vi "centerFilter.vi"(0 "Image In":T2, 1 "Color Mode (Color Threshold 1)":u16(ring) items=["RGB", "HSL", "HSV", "HSI"], 2 "Red or Hue Range (Color Threshold 1)":cluster{"Lower value":i32, "Upper value":i32}={"Lower value"=0, "Upper value"=12}, 3 "Green or Sat Range (Color Threshold 1)":cluster{"Lower value":i32, "Upper value":i32}={"Lower value"=24, "Upper value"=255}, 5 "Blue\nBlue or Sat Range (Color Threshold 1)":cluster{"Lower value":i32, "Upper value":i32}={"Lower value"=24, "Upper value"=255}, 7 "error in":errorcluster) -> (20 "Image Out":T2, 21 "Centroid (Centroid 1)":cluster{"X Centroid":sgl, "Y Centroid":sgl} {"Y Centroid" format="%.2f"; "X Centroid" format="%.2f"}, 22 "Calibrated Centroid (Centroid 1)":cluster{"X Centroid":sgl, "Y Centroid":sgl} {"Y Centroid" format="%.2f"; "X Centroid" format="%.2f"}, 23 "Particle Reports (Pixels)":T1(array[cluster]) {"Orientation" format="%.2f"; "Dimensions"."Height" format="%.2f"; "Dimensions"."Width" format="%.2f"; "Center of Mass"."Y" format="%.2f"; "Center of Mass"."X" format="%.2f"; "Bounding Rect"."Bottom" format="%.2f"; "Bounding Rect"."Right" format="%.2f"; "Bounding Rect"."Top" format="%.2f"; "Bounding Rect"."Left" format="%.2f"; "Number of Holes" format="%.2f"; "Area" format="%.2f"}, 24 "Number of Particles":i32, 27 "error out":errorcluster)   [LabVIEW 2020]
uses:
  <vilib>/vision/Image Controls.llb/IMAQ Image.ctl
  <vilib>/vision/NI_Vision_Development_Module.lvlib
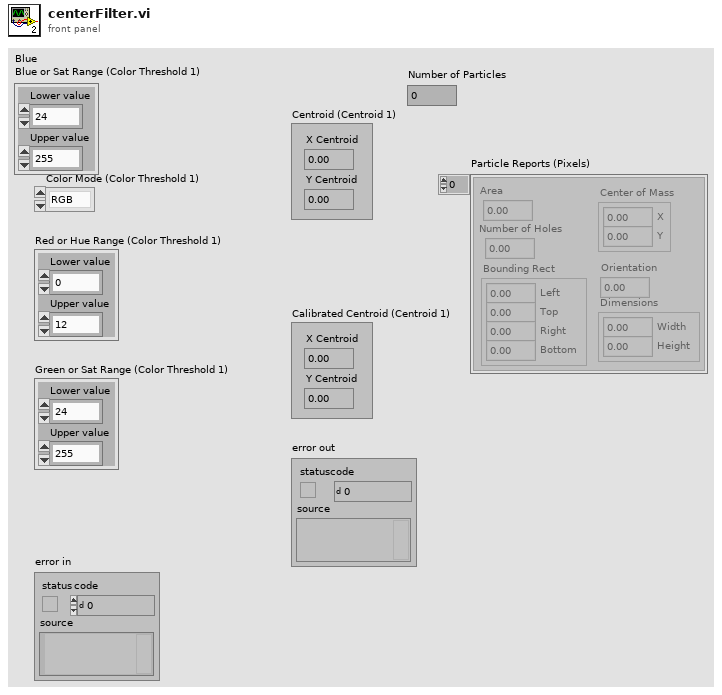
[diagram p1: front panel]
types:
  T1 = cluster{"Area":dbl, "Number of Holes":dbl, "Bounding Rect":cluster{"Left":dbl, "Top":dbl, "Right":dbl, "Bottom":dbl}, "Center of Mass":cluster{"X":dbl, "Y":dbl}, "Orientation":dbl, "Dimensions":cluster{"Width":dbl, "Height":dbl}}[]
  T2 = typedef "IMAQ Image.ctl" = refnum<image>
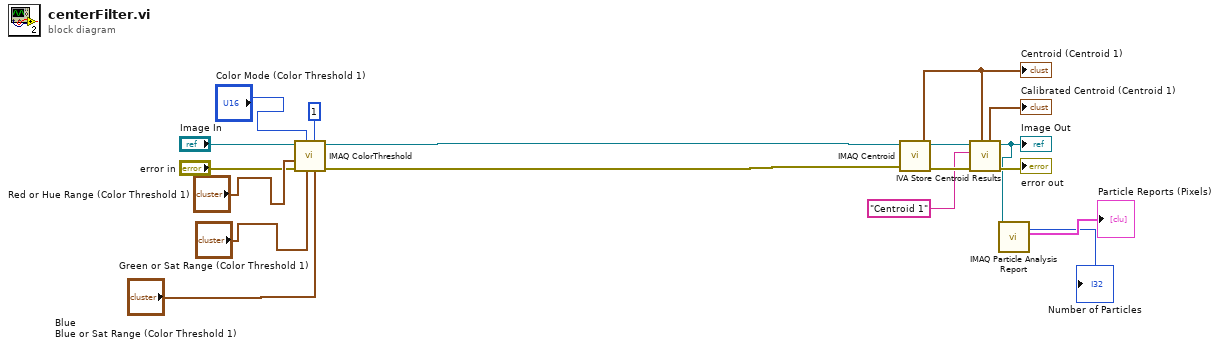
[diagram p0: block diagram]
diagram:
  n1 = call "IMAQ ColorThreshold"("Blue or Luma or Val or Inten Range"="Blue\nBlue or Sat Range (Color Threshold 1)", "Replace Value"=1, "Green or Sat Range"="Green or Sat Range (Color Threshold 1)", "Color Mode"="Color Mode (Color Threshold 1)", "error in (no error)"="error in", "Red or Hue Range"="Red or Hue Range (Color Threshold 1)", "Image Src"="Image In") -> ("error out"=w1:errorcluster, "Image Dst Out"=w2:T2)  [unwired: 1 in, 2 out]
  n2 = call "IMAQ Centroid"("error in (no error)"=w1, "Image"=w2) -> ("error out"=w11:errorcluster, "Centroid"=w8:cluster{"X Centroid":sgl, "Y Centroid":sgl})  [unwired: 1 in, 1 out]
  "Centroid (Centroid 1)" <- w8
  n3 = call <vilib>:"IVA Store Centroid Results.vi"("Centroid in"=w8, "error in (no error)"=w11, "Step Name"="Centroid 1", "Image in"=w2) -> ("error out"=→"error out":errorcluster, "Image dup"=w6:T2, "Calibrated Centroid"=→"Calibrated Centroid (Centroid 1)":cluster{"X":sgl, "Y":sgl})  [unwired: 5 out]
  "Image Out" <- w6
  n4 = call "IMAQ Particle Analysis Report"("Image"=w6) -> ("Particle Reports (Pixels)"=→"Particle Reports (Pixels)":T1, "Number of Particles"=→"Number of Particles":i32)  [unwired: 5 in, 4 out]
